vi "ex_6_odczyt_z_pliku_blednie.vi"() -> ()   [LabVIEW 2020]
uses:
  #typedef_Product.ctl
panel:
  out "Array 4":string[](array[string])
  out "Array 3":string[](array[string])
  out "Array 2":i32[](array[numeric])
  in  "Array":T1[](array[typedef])
  out "text":string
  in  "Path":path
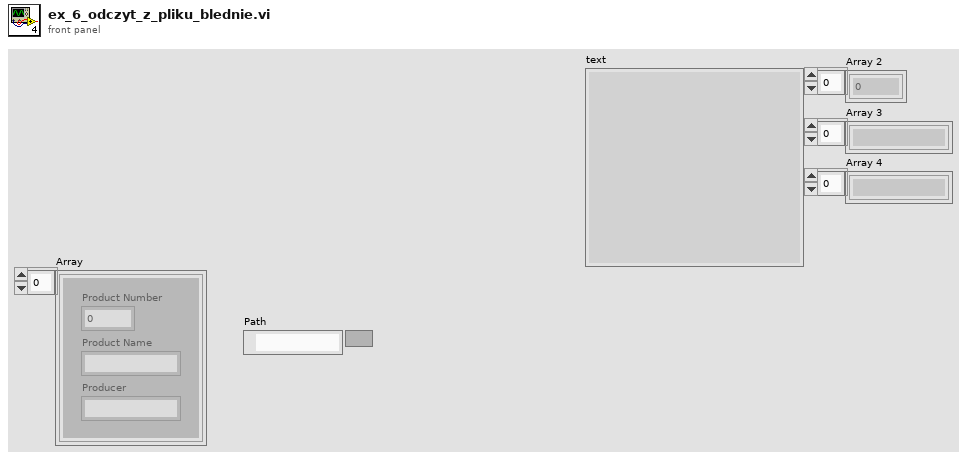
[diagram p1: front panel]
types:
  T1 = typedef "#typedef_Product.ctl" = cluster{"Product Number":i32, "Product Name":string, "Producer":string}
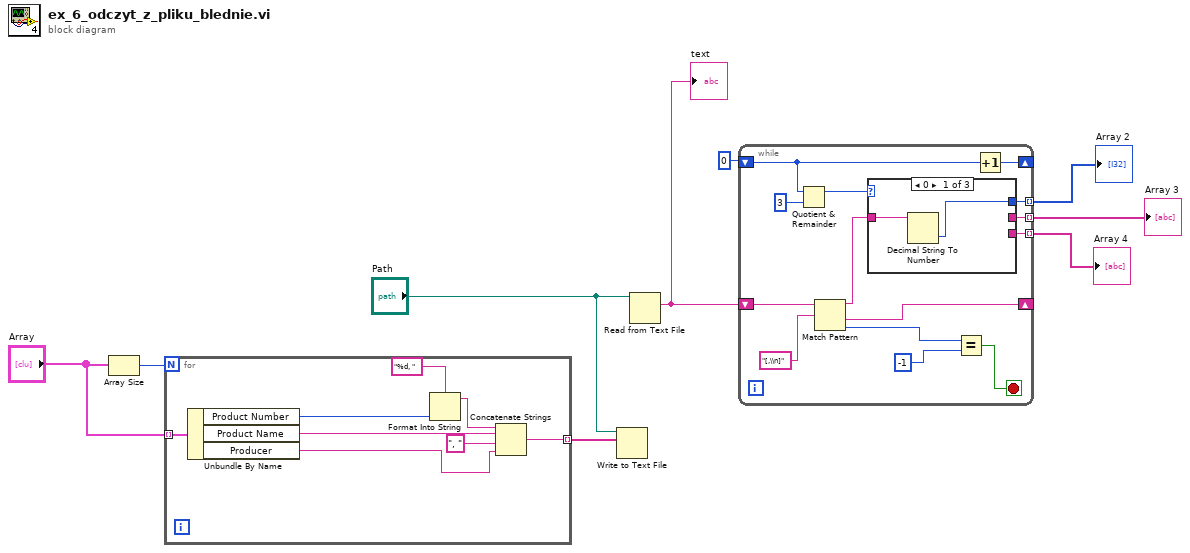
[diagram p0: block diagram]
diagram:
  n1 = Array Size(array="Array") -> (size(s)=w6:i32)
  n2 = for {
    N: w6 -> [_]
    tunnel: "Array" -> [w17] mode=indexing
    tunnel: [w10] -> w8 mode=indexing
    n3 = Unbundle By Name(w17) -> ("Product Number"=w16:i32, "Product Name"=w13:string, "Producer"=w11:string)
    n4 = Format Into String(format string="%d, ", w16) -> (resulting string=w14:string)  [unwired: 2 in, 1 out]
    n5 = Concatenate Strings(w14, w13, ", " ("string"), w11) -> (w10:string)
  }
  n6 = Write to Text File(file (use dialog)="Path", text=w8) -> ()  [unwired: 2 in, 3 out]
  n7 = Read from Text File(file (use dialog)="Path") -> (text=w9:string)  [unwired: 3 in, 3 out]
  "text" <- w9
  n8 = while {
    shift-right: [w27] -> _
    shift-left: w9 -> [w26]
    shift-right: [w25] -> _
    shift-left: 0 -> [w24]
    tunnel: [w20] -> w3 mode=indexing
    tunnel: [w19] -> w2 mode=indexing
    tunnel: [w18] -> w1 mode=indexing
    stop <- w28 stop-if-true
    n9 = Quotient & Remainder(x=w24, y=3) -> (x-y*floor(x/y)=w22:i32)  [unwired: 1 out]
    n10 = Match Pattern(string=w26, regular expression="[,\\n]") -> (before substring=w21:string, after substring=w27:string, offset past match=w30:i32)  [unwired: 1 in, 1 out]
    n11 = case shown="0" w22 {
      tunnel: w21 -> [w33 w34 w35]
      tunnel: [w32 _ _] -> w20
      tunnel: [_ w34 _] -> w19
      tunnel: [_ _ w35] -> w18
      frame 0 {
        n12 = Decimal String To Number(string=w33) -> (number=w32:i32)  [unwired: 2 in, 1 out]
      }
      frame 1 {
      }
      frame 2 {
      }
    }
    n13 = Equal?(x=w30, y=-1) -> (x = y?=w28:bool)
    n14 = Increment(x=w24) -> (x+1=w25:i32)
  }
  "Array 2" <- w3
  "Array 3" <- w2
  "Array 4" <- w1
